vi "Olympus Command.vi"(8 "error in (no error)":errorcluster {"code" format="%.0x"}, 9 "Command string":string, 10 "Device Number (1)":i32=1, 11 "VISA Resource Name":refnum<visa-resource-name>) -> (0 "error out":errorcluster {"code" format="%.0x"}, 2 "Result":string, 3 "VISA Resource Name Out":refnum<visa-resource-name>)   [LabVIEW 2020, in "Olympus IX BX Series.lvlib"]
doc: "This VI create correct syntax of command for instrument and send it into instrument.\nWhen query command is specified VI return parameter of command."
uses:
  Olympus IX BX Series.lvlib
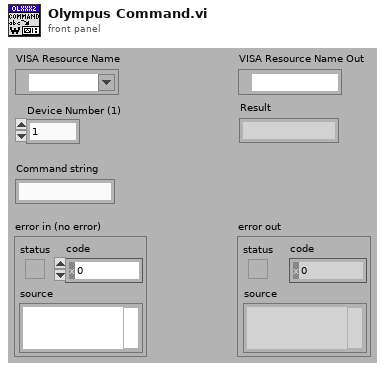
[diagram p1: front panel]
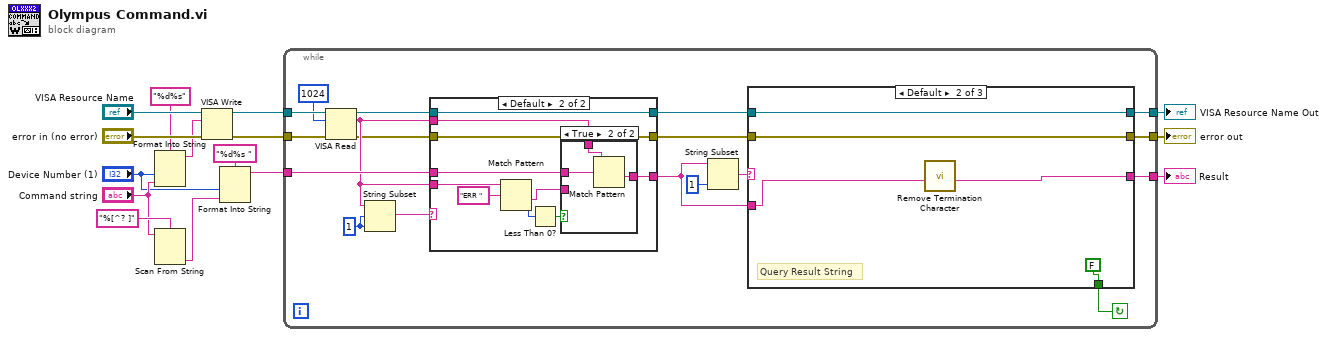
[diagram p0: block diagram]
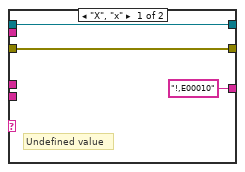
[diagram p2: hidden frame]
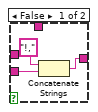
[diagram p3: hidden frame]
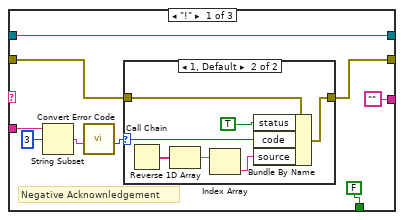
[diagram p4: hidden frame]
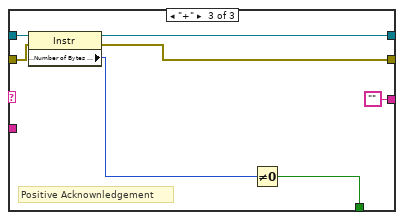
[diagram p6: hidden frame]
diagram:
  n1 = Format Into String(format string="%d%s", "Device Number (1)", "Command string") -> (resulting string=w9:string)  [unwired: 2 in, 1 out]
  n2 = Scan From String(format string="%[^? ]", input string="Command string") -> (output 1=w6:string)  [unwired: 3 in, 3 out]
  n3 = VISA Write(VISA resource name="VISA Resource Name", write buffer=w9, error in (no error)="error in (no error)") -> (VISA resource name out=w11:refnum<visa-resource-name>, error out=w12:errorcluster)  [unwired: 1 out]
  n4 = Format Into String(format string="%d%s ", "Device Number (1)", w6) -> (resulting string=w4:string)  [unwired: 2 in, 1 out]
  n5 = while {
    tunnel: w12 -> [w33]
    tunnel: w11 -> [w32]
    tunnel: w4 -> [w30]
    tunnel: [w29] -> w3
    tunnel: [w28] -> w2
    tunnel: [w27] -> w1
    stop <- w23 continue-if-true
    w22 = 1 ("length (rest)")
    n6 = VISA Read(VISA resource name=w32, byte count=u32 1024, error in (no error)=w33) -> (VISA resource name out=w19:refnum<visa-resource-name>, read buffer=w20:string, error out=w17:errorcluster)  [unwired: 1 out]
    n7 = String Subset(string=w20, offset (0)=w22, length (rest)=w22) -> (substring=w21:string)
    n8 = case shown="Default" w21 {
      tunnel: w30 -> [_ w46]
      tunnel: ["!,E00010" w45] -> w26
      tunnel: w20 -> [_ w40]
      tunnel: w20 -> [_ w39]
      tunnel: w19 -> [w36 w38]
      tunnel: [w36 w38] -> w18
      tunnel: w17 -> [w35 w37]
      tunnel: [w35 w37] -> w16
      frame "X", "x" {
        # "Undefined value"
      }
      frame Default {
        n9 = Match Pattern(string=w39, regular expression="ERR ") -> (after substring=w41:string, offset past match=w43:i32)  [unwired: 1 in, 2 out]
        n10 = Less Than 0?(x=w43) -> (x < 0?=w42:bool)
        n11 = case shown="True" w42 {
          tunnel: w46 -> [_ w52]
          tunnel: [w48 w51] -> w45
          tunnel: w40 -> [_ w50]
          tunnel: w41 -> [w49 _]
          frame False {
            n12 = Concatenate Strings("!," ("string"), w49) -> (w48:string)
          }
          frame True {
            n13 = Match Pattern(string=w50, regular expression=w52) -> (after substring=w51:string)  [unwired: 1 in, 3 out]
          }
        }
      }
    }
    n14 = String Subset(string=w26, length (rest)=1 ("length (rest)")) -> (substring=w25:string)  [unwired: 1 in]
    n15 = case shown="Default" w25 {
      tunnel: w16 -> [w55 w74 w79]
      tunnel: [w54 w74 w77] -> w29
      tunnel: w16 -> [_ _ _]
      tunnel: [w60 w73 w78] -> w28
      tunnel: w18 -> [w60 w73 w80]
      tunnel: ["" w71 ""] -> w27
      tunnel: w26 -> [w59 w72 _]
      tunnel: [FALSE FALSE w75] -> w23
      frame "!" {
        # "Negative Acknownledgement"
        n16 = String Subset(string=w59, offset (0)=3) -> (substring=w57:string)  [unwired: 1 in]
        n17 = call "Convert Error Code.vi"("Error String"=w57) -> ("VISA Error Code"=w56:i32)  [unwired: 10 in]
        n18 = case shown="1, Default" w56 {
          selector: w56 -> [_ w66]
          tunnel: w55 -> [w62 w67]
          tunnel: [w62 w63] -> w54
          frame 0 {
          }
          frame 1, Default {
            n19 = Call Chain() -> (call chain=w69:string[])
            n20 = Reverse 1D Array(array=w69) -> (reversed array=w68:string[])
            n21 = Index Array(array=w68) -> (element=w65:string)  [unwired: 1 in]
            n22 = Bundle By Name(cluster=w67, "status"=TRUE, "code"=w66, "source"=w65) -> (w63:errorcluster)
          }
        }
      }
      frame Default {
        # "Query Result String"
        n23 = call "Remove Termination Character.vi"("Input string"=w72) -> ("String before CR+LF"=w71:string)  [unwired: 10 in]
      }
      frame "+" {
        # "Positive Acknownledgement"
        n24 = property class="Instr"(reference=w80, error in=w79) -> (reference out=w78:refnum<visa-resource-name>, error out=w77:errorcluster, "Serial Settings:Number of Bytes at Serial Port"=w76:u32)
        n25 = Not Equal To 0?(x=w76) -> (x != 0?=w75:bool)
      }
    }
  }
  "VISA Resource Name Out" <- w2
  "error out" <- w3
  "Result" <- w1
